vi "GearLift.vi"(11 "Gear Up":bool) -> ()   [LabVIEW 2016]
uses:
  <vilib>/Rock Robotics/WPI/Solenoid/Deprecated/WPI_SolenoidSetBool.vi
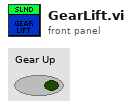
[diagram p1: front panel]
types:
  T1 = typedef "WPI_SolenoidDevRef.ctl" = cluster{"DevStatus":errorcluster, "Pneumatics Control Module":u8, "Forward Solenoid Channel":T2, "Reverse Solenoid Channel":T2}
  T2 = typedef "WPI_SolenoidChannel.ctl" = enum8{"Solenoid 0", "Solenoid 1", "Solenoid 2", "Solenoid 3", "Solenoid 4", "Solenoid 5", "Solenoid 6", "Solenoid 7", "Invalid"}
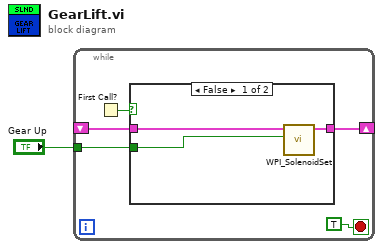
[diagram p0: block diagram]
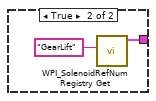
[diagram p2: hidden frame]
diagram:
  n1 = while {
    tunnel: "Gear Up" -> [w2]
    shift-right: [w4] -> _
    shift-left: _ -> [w3]
    stop <- TRUE stop-if-true
    n2 = First Call?() -> (First Call?: T/F=w6:bool)
    n3 = case shown="False" w6 {
      tunnel: [w8 w10] -> w4
      tunnel: w3 -> [w9 _]
      tunnel: w2 -> [w7 _]
      frame False {
        n4 = call-poly <vilib>:"WPI_SolenoidSet.vi"("Value"=w7, "SolenoidDevRef"=w9) -> ("SolenoidDevRef"=w8:T1)  [unwired: 8 in, 1 out]
      }
      frame True {
        n5 = call <vilib>:"WPI_SolenoidRefNum Registry Get.vi"("refnum name"="GearLift") -> ("SolenoidDevRef"=w10:T1)  [unwired: 9 in, 1 out]
      }
    }
  }
